vi "_Init Res.vi"(8 "error in (no error)":errorcluster, 10 "WebView2 Control":refnum<k24>, 11 "WebView2 Control in":refnum<class "WebView2 Control.lvclass">) -> (0 "error out":errorcluster, 3 "WebView2 Control out":refnum<class "WebView2 Control.lvclass">)   [LabVIEW 2025, in "WebView2.lvlib" / "WebView2 Control.lvclass"]
uses:
  WebView2 Control.lvclass
  E:/Labview/LV 2023/PPL/PPL Builder/Libs/LV-WebView2/Source/Libs/Microsoft.Web.WebView2.WinForms.dll
  Libs/Microsoft.Web.WebView2.WinForms.dll
  Source Changed Event Data.ctl
  Events.ctl
  Navigation Event Data.ctl
  Web Message Received Event Data.ctl
  Navigation Start Event Data.ctl
  WebView2 Event Filter Interface/WebView2 Event Filter Interface.lvclass
  New Window Event Data.ctl
  Content Loading Event Data.ctl
  <vilib>/Utility/sysdir.llb/System Directory Type.ctl
  Res.ctl
  WebView2 Control.lvclass/WebView2 Control.ctl
  E:/Labview/LV 2023/PPL/PPL Builder/Libs/LV-WebView2/Source/Libs/Microsoft.Web.WebView2.Core.dll
  Libs/Microsoft.Web.WebView2.Core.dll
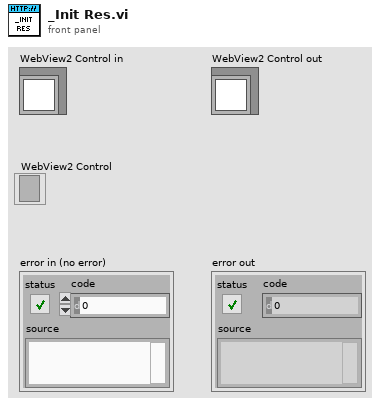
[diagram p1: front panel]
types:
  T1 = typedef "WebView2.lvlib/WebView2 Control.lvclass/New Window Event Data.ctl" = cluster{"IsUserInitiated":bool, "Name":string, "Uri":string, "Filter":refnum<class "WebView2 Event Filter Interface.lvclass">, "OriginalSourceFrameInfo":refnum<k24>, "WindowFeatures":refnum<k24>}
  T2 = typedef "WebView2.lvlib/WebView2 Control.lvclass/Res.ctl" = cluster{"WebView2":refnum<k24>, "Webview2 Core":refnum<k24>, "event callback":refnum<k27>, "Environment":refnum<k24>}
  T3 = typedef "WebView2.lvlib/WebView2 Control.lvclass/Navigation Start Event Data.ctl" = cluster{"AdditionalAllowedFrameAncestors":string, "IsRedirected":bool, "IsUserInitiated":bool, "NavigationId":u64, "NavigationKind":i32, "Uri":string, "Headers":cluster{"Key":string, "Value":string}[], "Event Filter":refnum<class "WebView2 Event Filter Interface.lvclass">}
  T4 = typedef "WebView2.lvlib/WebView2 Control.lvclass/Navigation Event Data.ctl" = cluster{"HttpStatusCode":i32, "IsSuccess":bool, "NavigationId":u64, "WebErrorStatus":i32}
  T5 = typedef "System Directory Type.ctl" = i32
  T6 = typedef "WebView2.lvlib/WebView2 Control.lvclass/Web Message Received Event Data.ctl" = cluster{"Source":string, "WebMessageAsJson":string, "AdditionalObjects":refnum<k24>}
  T7 = typedef "WebView2.lvlib/WebView2 Control.lvclass/Events.ctl" = cluster{"Navigation Complete Event":refnum<user-event>, "Source Changed Event":refnum<user-event>, "Document Title Changed Event":refnum<user-event>, "Status Bar Text Changed":refnum<user-event>, "Web Message Received":refnum<user-event>, "Window Close Requested":refnum<user-event>, "DOM Loaded":refnum<user-event>, "Navigation Started Event":refnum<user-event>, "New Window Requested Event":refnum<user-event>, "Content Loading Event":refnum<user-event>}
  T8 = typedef "WebView2.lvlib/WebView2 Control.lvclass/Source Changed Event Data.ctl" = cluster{"Source":string, "IsNewDocument":bool}
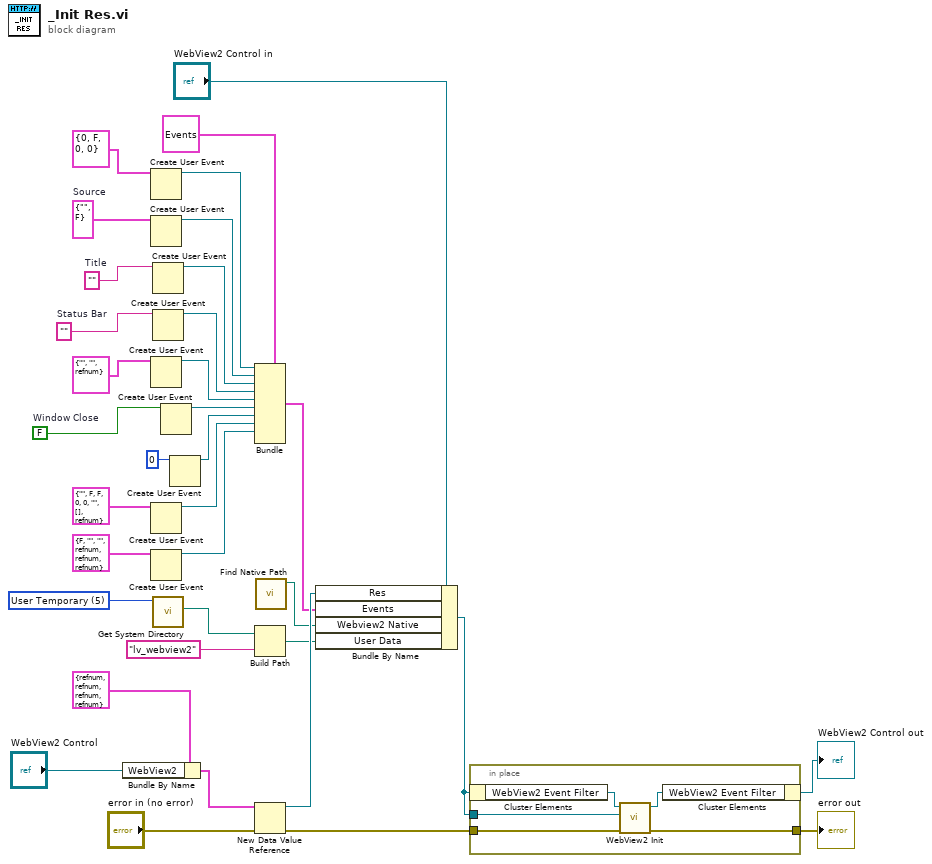
[diagram p0: block diagram]
diagram:
  w21 = T5 5 items=["User Home"=0, "User Desktop"=1, "User Documents"=2, "User Application Data"=3, "User Preferences"=4, "User Temporary"=5, "Public Documents"=6, "Public Application Data"=7, "Public Preferences"=8, "Public Cache"=13, "System Core Libraries"=9, "System Installed Libraries"=10, "Application Files"=11, "Boot Volume Root"=12] ("system directory type")
  w18 = FALSE  # Window Close
  w15 = ""  # Status Bar
  w9 = ""  # Title
  w8 = T8 {"Source"="", "IsNewDocument"=FALSE}  # Source
  n1 = Bundle By Name(cluster=T2 {"WebView2"=refnum, "Webview2 Core"=refnum, "event callback"=refnum, "Environment"=refnum} ("output cluster"), "WebView2"="WebView2 Control") -> (w32:T2)
  n2 = Create User Event(user event datatype=T4 {"HttpStatusCode"=0, "IsSuccess"=FALSE, "NavigationId"=0, "WebErrorStatus"=0} ("output cluster")) -> (user event=w13:refnum<user-event>)  [unwired: 1 in, 1 out]
  n3 = Create User Event(user event datatype=w8) -> (user event=w14:refnum<user-event>)  [unwired: 1 in, 1 out]
  n4 = Create User Event(user event datatype=T6 {"Source"="", "WebMessageAsJson"="", "AdditionalObjects"=refnum} ("output cluster")) -> (user event=w17:refnum<user-event>)  [unwired: 1 in, 1 out]
  n5 = Create User Event(user event datatype=T3 {"AdditionalAllowedFrameAncestors"="", "IsRedirected"=FALSE, "IsUserInitiated"=FALSE, "NavigationId"=0, "NavigationKind"=0, "Uri"="", "Headers"=[], "Event Filter"=refnum} ("Nav Started Event")) -> (user event=w29:refnum<user-event>)  [unwired: 1 in, 1 out]
  n6 = Create User Event(user event datatype=T1 {"IsUserInitiated"=FALSE, "Name"="", "Uri"="", "Filter"=refnum, "OriginalSourceFrameInfo"=refnum, "WindowFeatures"=refnum} ("cluster")) -> (user event=w5:refnum<user-event>)  [unwired: 1 in, 1 out]
  n7 = Create User Event(user event datatype=w9) -> (user event=w12:refnum<user-event>)  [unwired: 1 in, 1 out]
  n8 = Create User Event(user event datatype=w15) -> (user event=w16:refnum<user-event>)  [unwired: 1 in, 1 out]
  n9 = call <vilib>:"Get System Directory.vi"("system directory type"=w21) -> ("system directory"=w22:path)  [unwired: 10 in]
  n10 = Create User Event(user event datatype=w18) -> (user event=w19:refnum<user-event>)  [unwired: 1 in, 1 out]
  n11 = Create User Event(user event datatype=u64 0 ("NavigationId")) -> (user event=w26:refnum<user-event>)  [unwired: 1 in, 1 out]
  n12 = Bundle(cluster=T7 {"Navigation Complete Event"=refnum, "Source Changed Event"=refnum, "Document Title Changed Event"=refnum, "Status Bar Text Changed"=refnum, "Web Message Received"=refnum, "Window Close Requested"=refnum, "DOM Loaded"=refnum, "Navigation Started Event"=refnum, "New Window Requested Event"=refnum, "Content Loading Event"=refnum} ("Cluster"), "Navigation Complete Event"=w13, "Source Changed Event"=w14, "Document Title Changed Event"=w12, "Status Bar Text Changed"=w16, "Web Message Received"=w17, "Window Close Requested"=w19, "DOM Loaded"=w26, "Navigation Started Event"=w29, "New Window Requested Event"=w5) -> (w11:T7)  [unwired: 1 in]
  n13 = Build Path(base path=w22, name or relative path="lv_webview2") -> (appended path=w25:path)
  n14 = New Data Value Reference(data value=w32, error in="error in (no error)") -> (data value reference=w33:refnum<data-value>, error out=w2:errorcluster)
  n15 = call "Find Native Path.vi"() -> ("path"=w24:path)  [unwired: 11 in]
  n16 = Bundle By Name(cluster="WebView2 Control in", "Res"=w33, "Events"=w11, "Webview2 Native"=w24, "User Data"=w25) -> (w3:refnum<class "WebView2 Control.lvclass">)
  n17 = in-place {
    in-place-border: w3 -> [w39]
    in-place-border: w2 -> [w38]
    in-place-border: [w36] -> w1
    n18 = in-place-cluster #1(w3) -> ("WebView2 Event Filter"=w40:refnum<class "WebView2 Event Filter Interface.lvclass">)
    n19 = call-dynamic "WebView2 Init.vi"("error in (no error)"=w38, "WebView2 Control"=w39, "WebView2 Event Filter Interface in"=w40) -> ("error out"=w36:errorcluster, "WebView2 Event Filter Interface out"=w37:refnum<class "WebView2 Event Filter Interface.lvclass">)  [unwired: 7 in]
    n20 = in-place-cluster #1("WebView2 Event Filter"=w37) -> (→"WebView2 Control out":refnum<class "WebView2 Control.lvclass">)
  }
  "error out" <- w1
